vi "LaserRestartTextScript.vi"(8 "ErrorIn":errorcluster) -> (0 "ErrorOut":errorcluster)   [LabVIEW 2012]
panel:
  out "CommandIn":string
  out "CommandOut":string
  out "Local Queue Response":string="Exit Idle Loop"
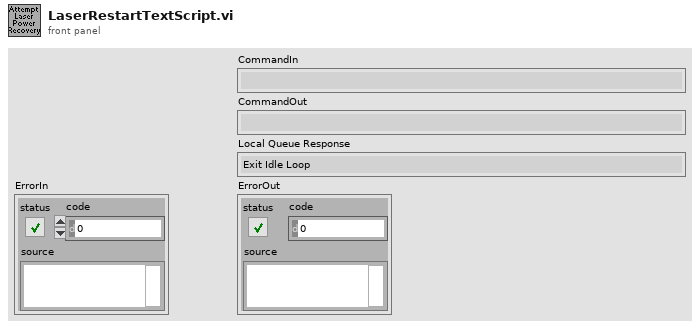
[diagram p1: front panel]
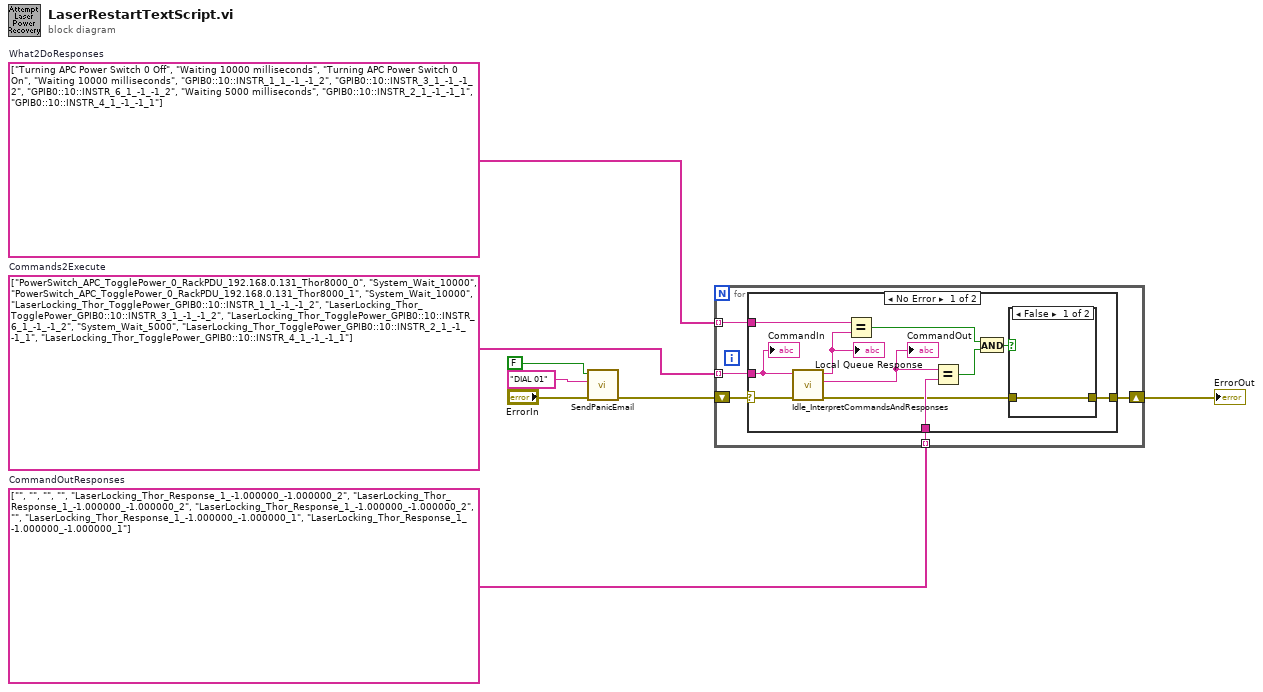
[diagram p0: block diagram]
diagram:
  w7 = string[] ["Turning APC Power Switch 0 Off", "Waiting 10000 milliseconds", "Turning APC Power Switch 0 On", "Waiting 10000 milliseconds", "GPIB0::10::INSTR_1_1_-1_-1_2", "GPIB0::10::INSTR_3_1_-1_-1_2", "GPIB0::10::INSTR_6_1_-1_-1_2", "Waiting 5000 milliseconds", "GPIB0::10::INSTR_2_1_-1_-1_1", "GPIB0::10::INSTR_4_1_-1_-1_1"]  # What2DoResponses
  w6 = string[] ["", "", "", "", "LaserLocking_Thor_Response_1_-1.000000_-1.000000_2", "LaserLocking_Thor_Response_1_-1.000000_-1.000000_2", "LaserLocking_Thor_Response_1_-1.000000_-1.000000_2", "", "LaserLocking_Thor_Response_1_-1.000000_-1.000000_1", "LaserLocking_Thor_Response_1_-1.000000_-1.000000_1"]  # CommandOutResponses
  w5 = string[] ["PowerSwitch_APC_TogglePower_0_RackPDU_192.168.0.131_Thor8000_0", "System_Wait_10000", "PowerSwitch_APC_TogglePower_0_RackPDU_192.168.0.131_Thor8000_1", "System_Wait_10000", "LaserLocking_Thor_TogglePower_GPIB0::10::INSTR_1_1_-1_-1_2", "LaserLocking_Thor_TogglePower_GPIB0::10::INSTR_3_1_-1_-1_2", "LaserLocking_Thor_TogglePower_GPIB0::10::INSTR_6_1_-1_-1_2", "System_Wait_5000", "LaserLocking_Thor_TogglePower_GPIB0::10::INSTR_2_1_-1_-1_1", "LaserLocking_Thor_TogglePower_GPIB0::10::INSTR_4_1_-1_-1_1"]  # Commands2Execute
  n1 = call "SendPanicEmail.vi"("ErrorIn"="ErrorIn", "DIALNumber"="DIAL 01", "TypeOfEmail"=FALSE) -> ("ErrorOut"=w3:errorcluster)  [unwired: 8 in]
  n2 = for {
    shift-right: [w13] -> w8
    shift-left: w3 -> [w12]
    tunnel: w5 -> [w11] mode=indexing
    tunnel: w7 -> [w10] mode=indexing
    tunnel: w6 -> [w9] mode=indexing
    n3 = case shown="No Error" w12 {
      selector: w12 -> [w24 w27]
      tunnel: [w15 w27] -> w13
      tunnel: w11 -> [w23 _]
      tunnel: w10 -> [w22 _]
      tunnel: w9 -> [w18 _]
      frame No Error {
        n4 = call "Idle_InterpretCommandsAndResponses.vi"("ErrorIn"=w24, "Input Command"=w23) -> ("ErrorOut"=w16:errorcluster, "Command Out"=w14:string, "What to Do"=w21:string)  [unwired: 6 in, 1 out]
        "Local Queue Response" <- w21
        "CommandOut" <- w14
        n5 = Equal?(x=w22, y=w21) -> (x = y?=w20:bool)
        n6 = Equal?(x=w14, y=w18) -> (x = y?=w19:bool)
        n7 = And(x=w20, y=w19) -> (x .and. y?=w17:bool)
        n8 = case shown="False" w17 {
          tunnel: w16 -> [w25 w26]
          tunnel: [w25 w26] -> w15
          frame False {
          }
          frame True {
          }
        }
        "CommandIn" <- w23
      }
      frame Error {
      }
    }
  }
  "ErrorOut" <- w8
